vi "HumanExecute.vi"(8 "error in (no error)":errorcluster) -> (0 "error out":errorcluster)   [LabVIEW 2023]
doc: "Execute for Human\n\ninput:\n error in (cluster)\n\noutput:\n error out (cluster)"
uses:
  Arm/ArmPositionPreset.ctl
  Arm/ArmGamePiecePreset.ctl
  <vilib>/Rock Robotics/WPI/Joystick/XBox Buttons Indexer.ctl
  <vilib>/Rock Robotics/WPI/Joystick/XBox Axes Indexer.ctl
  <vilib>/Rock Robotics/WPI/ThirdParty/JAS_Junk/TrajLib/Timer_New.vi
  Claw/ClawGlobal.vi
  <vilib>/Utility/semaphor.llb/Obtain Semaphore Reference.vi
  <vilib>/Rock Robotics/WPI/ThirdParty/JAS_Junk/TrajLib/Timer_Reset.vi
  <vilib>/Rock Robotics/WPI/ThirdParty/JAS_Junk/TrajLib/Timer_Start.vi
  <vilib>/Rock Robotics/WPI/ThirdParty/JAS_Junk/TrajLib/Timer_HasPeriodPassedOnce.vi
  <vilib>/Rock Robotics/WPI/ThirdParty/JAS_Junk/TrajLib/Timer_Stop.vi
  <vilib>/Rock Robotics/WPI/ThirdParty/JAS_Junk/TrajLib/Trajectory_Library.lvlib
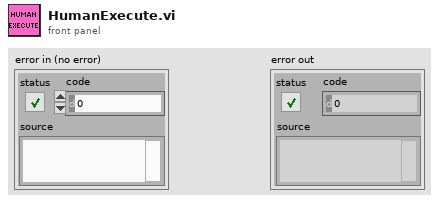
[diagram p1: front panel]
types:
  T1 = typedef "ArmPositionPreset.ctl" = enum16{"Upper", "Lower", "Middle", "Home", "Shelf", "Floor", "HalfFloor", "HalfHome"}
  T2 = typedef "ArmGamePiecePreset.ctl" = enum16{"Cube", "Cone"}
  T3 = typedef "XBox Buttons Indexer.ctl" = enum16{"A", "B", "X", "Y", "Left Bumper", "Right Bumper", "Back", "Start", "Left Joystick", "Right Joystick"}
  T4 = typedef "XBox Axes Indexer.ctl" = enum16{"Left X", "Left Y", "Left Trigger", "Right Trigger", "Right X", "Right Y"}
  T5 = typedef "WPI_JoystickDevRef.ctl" = cluster{"Device":T6}
  T6 = typedef "WPI_JoystickDeviceEnum.ctl" = enum16{"USB 0", "USB 1", "USB 2", "USB 3", "USB 4", "USB 5"}
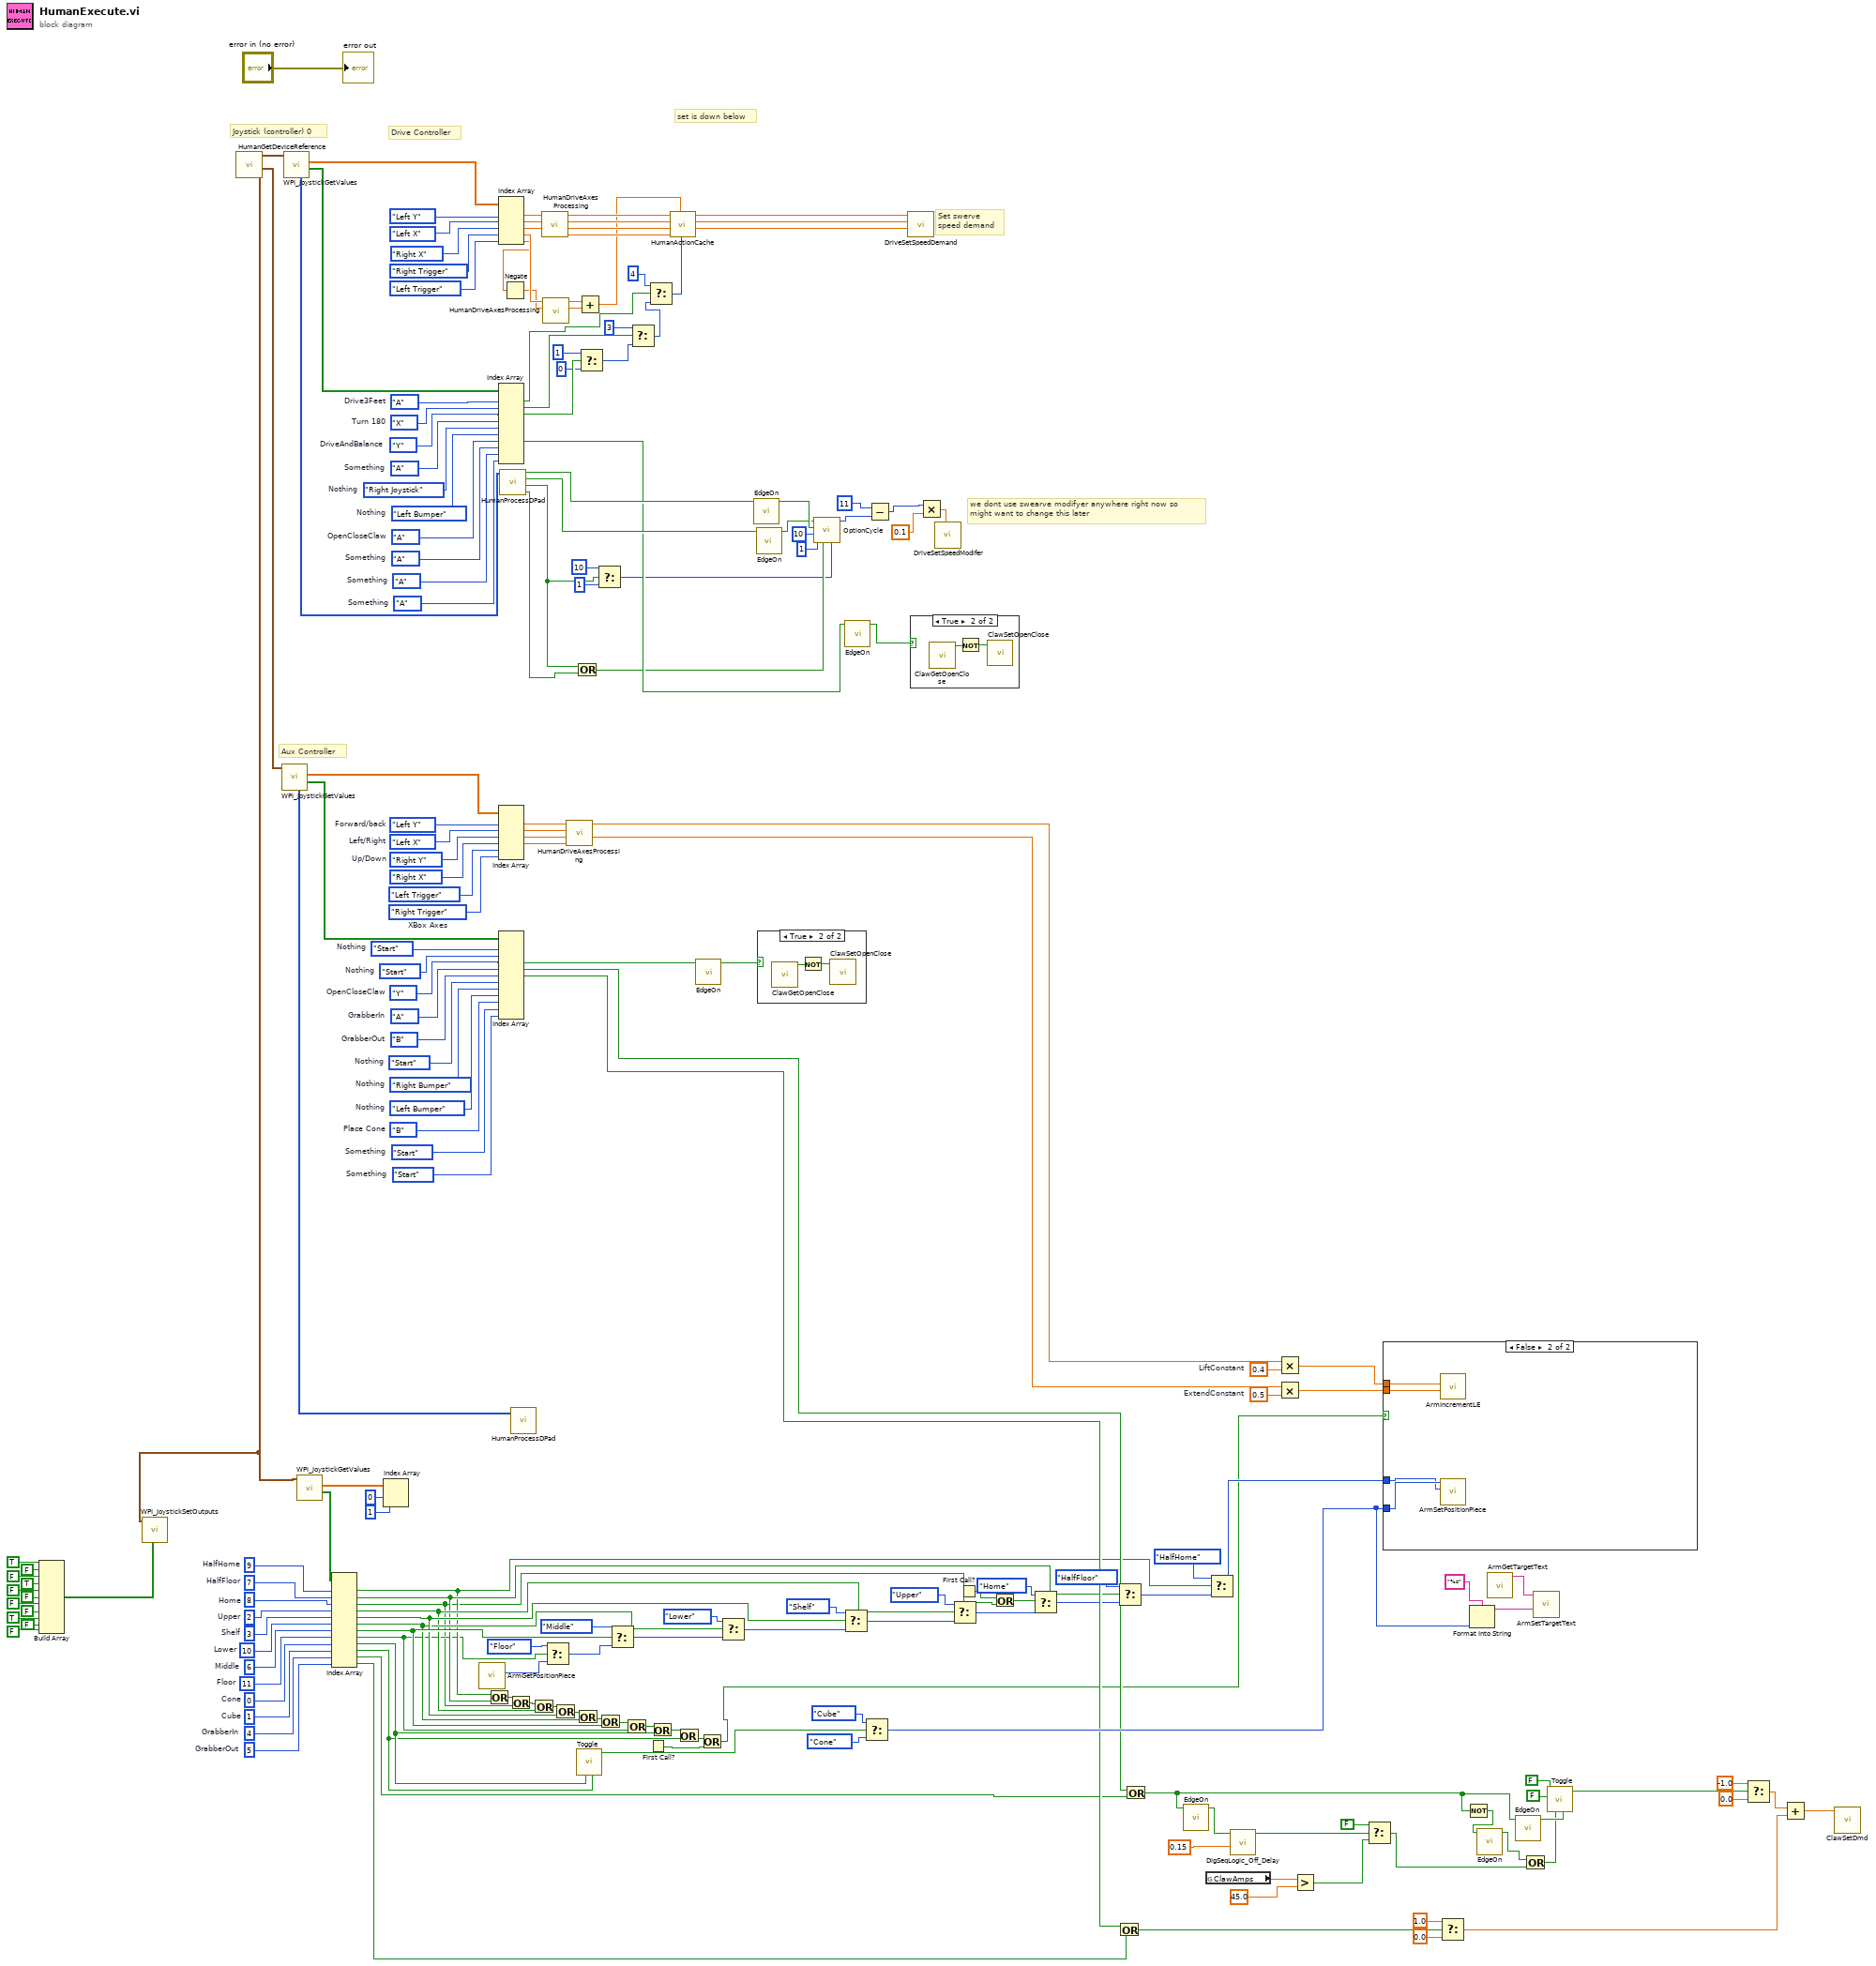
[diagram p0: block diagram]
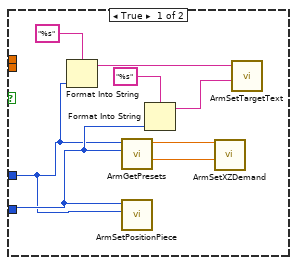
[diagram p3: hidden frame]
diagram:
  w58 = 9  # HalfHome
  w59 = 7  # HalfFloor
  w96 = 8  # Home
  w103 = 0.4  # LiftConstant
  w104 = 0.5  # ExtendConstant
  w116 = 5  # GrabberOut
  w117 = 4  # GrabberIn
  w118 = 1  # Cube
  w119 = 0  # Cone
  w120 = 11  # Floor
  w121 = 6  # Middle
  w122 = 10  # Lower
  w123 = 3  # Shelf
  w124 = 2  # Upper
  w135 = XBox_Buttons_Indexer."Start"  # Something
  w136 = XBox_Buttons_Indexer."Start"  # Something
  w137 = XBox_Buttons_Indexer."B"  # Place Cone
  w138 = XBox_Buttons_Indexer."Left Bumper"  # Nothing
  w139 = XBox_Buttons_Indexer."Right Bumper"  # Nothing
  w140 = XBox_Buttons_Indexer."Start"  # Nothing
  w145 = XBox_Buttons_Indexer."B"  # GrabberOut
  w148 = XBox_Buttons_Indexer."A"  # GrabberIn
  w149 = XBox_Buttons_Indexer."Y"  # OpenCloseClaw
  w150 = XBox_Buttons_Indexer."Start"  # Nothing
  w151 = XBox_Buttons_Indexer."Start"  # Nothing
  w141 = XBox_Axes_Indexer."Right Trigger"  # XBox Axes
  w144 = XBox_Axes_Indexer."Right Y"  # Up/Down
  w152 = XBox_Axes_Indexer."Left X"  # Left/Right
  w153 = XBox_Axes_Indexer."Left Y"  # Forward/back
  w179 = XBox_Buttons_Indexer."A"  # Something
  w180 = XBox_Buttons_Indexer."A"  # Something
  w181 = XBox_Buttons_Indexer."A"  # Something
  w182 = XBox_Buttons_Indexer."A"  # OpenCloseClaw
  w183 = XBox_Buttons_Indexer."Left Bumper"  # Nothing
  w190 = XBox_Buttons_Indexer."Right Joystick"  # Nothing
  w191 = XBox_Buttons_Indexer."A"  # Something
  w193 = XBox_Buttons_Indexer."Y"  # DriveAndBalance
  w194 = XBox_Buttons_Indexer."X"  # Turn 180
  w195 = XBox_Buttons_Indexer."A"  # Drive3Feet
  # "set is down below"
  # "we dont use swearve modifyer anywhere right now so\nmight want to change this later"
  # "Aux Controller"
  # "Set swerve\nspeed demand"
  # "Joystick (controller) 0"
  # "Drive Controller"
  n1 = Build Array(TRUE, FALSE ("element"), FALSE ("element"), TRUE ("element"), FALSE ("element"), FALSE ("element"), FALSE ("element"), FALSE ("element"), TRUE ("element"), FALSE ("element"), FALSE ("element")) -> (w173:bool[])
  n2 = call "HumanGetDeviceReference.vi"() -> ("ButtonBoard"=w174:T5, "Aux Joy"=w197:T5, "Driver Joy"=w198:T5)  [unwired: 9 in]
  n3 = call <vilib>:"WPI_JoystickSetOutputs.vi"("Outputs"=w173, "JoystickDevRef"=w174) -> ()  [unwired: 8 in, 2 out]
  n4 = call <vilib>:"WPI_JoystickGetValues.vi"("JoystickDevRef"=w197) -> ("Buttons"=w146:bool[], "Axes"=w147:dbl[], "POVs"=w134:i16[])  [unwired: 6 in, 2 out]
  n5 = call <vilib>:"WPI_JoystickGetValues.vi"("JoystickDevRef"=w198) -> ("Buttons"=w196:bool[], "Axes"=w202:dbl[], "POVs"=w192:i16[])  [unwired: 6 in, 2 out]
  n6 = call <vilib>:"WPI_JoystickGetValues.vi"("JoystickDevRef"=w174) -> ("Buttons"=w128:bool[], "Axes"=w127:dbl[])  [unwired: 6 in, 3 out]
  n7 = Index Array "Index Array"(array=w128, index #1=w58, index #2=w59, index #3=w96, index #4=w124, index #5=w123, index #6=w122, index #7=w121, index #8=w120, index #9=w119, index #10=w118, index #11=w117, index #12=w116) -> (element #1=w60:bool, element #2=w61:bool, element #3=w35:bool, element #4=w93:bool, element #5=w108:bool, element #6=w102:bool, element #7=w109:bool, element #8=w55:bool, element #9=w84:bool, element #10=w83:bool, element #11=w53:bool, element #12=w71:bool)
  n8 = Index Array "Index Array"(array=w127, index #1=0 ("index"), index #2=1 ("index")) -> ()  [unwired: 2 out]
  n9 = call "ArmGetPositionPiece.vi"() -> ("Position"=w54:T1)  [unwired: 10 in, 1 out]
  n10 = Or(x=w60, y=w61) -> (x .or. y?=w63:bool)
  n11 = Index Array(array=w202, index #1=XBox_Axes_Indexer."Left Y" ("XBox Axes"), index #2=XBox_Axes_Indexer."Left X" ("XBox Axes"), index #3=XBox_Axes_Indexer."Right X" ("XBox Axes"), index #4=XBox_Axes_Indexer."Right Trigger" ("XBox Axes"), index #5=XBox_Axes_Indexer."Left Trigger" ("XBox Axes")) -> (element #1=w188:dbl, element #2=w187:dbl, element #3=w186:dbl, element #4=w159:dbl, element #5=w158:dbl)
  n12 = Index Array(array=w196, index #1=w195, index #2=w194, index #3=w193, index #4=w191, index #5=w190, index #6=w183, index #7=w182, index #8=w181, index #9=w180, index #10=w179) -> (element #1=w2:bool, element #2=w164:bool, element #3=w184:bool, element #7=w175:bool)  [unwired: 6 out]
  n13 = Index Array(array=w147, index #1=w153, index #2=w152, index #3=w144, index #4=XBox_Axes_Indexer."Right X" ("XBox Axes"), index #5=XBox_Axes_Indexer."Left Trigger", index #6=w141) -> (element #1=w133:dbl, element #2=w132:dbl, element #3=w131:dbl, element #4=w130:dbl)  [unwired: 2 out]
  n14 = Index Array "Index Array"(array=w146, index #1=w151, index #2=w150, index #3=w149, index #4=w148, index #5=w145, index #6=w140, index #7=w139, index #8=w138, index #9=w137, index #10=w136, index #11=w135) -> (element #3=w107:bool, element #4=w70:bool, element #5=w69:bool)  [unwired: 8 out]
  n15 = call "HumanProcessDPad.vi"("POV"=w192) -> ("Right"=w171:bool, "Left"=w170:bool, "Down"=w177:bool, "Up"=w178:bool)  [unwired: 7 in]
  n16 = Negate(x=w158) -> (-x=w157:dbl)
  n17 = Or(x=w63, y=w35) -> (x .or. y?=w62:bool)
  n18 = call "HumanProcessDPad.vi"("POV"=w134) -> ()  [unwired: 7 in, 4 out]
  n19 = Or(x=w62, y=w93) -> (x .or. y?=w94:bool)
  n20 = call "HumanDriveAxesProcessing.vi"("Right Y"=w186, "Left X"=w187, "Left Y"=w188) -> ("Right X"=w185:dbl, "Right Y"=w154:dbl, "Left X"=w160:dbl, "Left Y"=w9:dbl)  [unwired: 5 in]
  n21 = call "HumanDriveAxesProcessing.vi"("Left X"=w157, "Left Y"=w159) -> ("Left X"=w155:dbl, "Left Y"=w156:dbl)  [unwired: 6 in, 2 out]
  n22 = Select(t=ArmPositionPreset."Floor" ("Position"), s=w55, f=w54) -> (s? t:f=w57:T1)
  n23 = Or(x=w94, y=w108) -> (x .or. y?=w112:bool)
  n24 = call "HumanDriveAxesProcessing.vi"("Right X"=w130, "Right Y"=w131, "Left X"=w132, "Left Y"=w133) -> ("Right Y"=w105:dbl, "Left Y"=w106:dbl)  [unwired: 4 in, 2 out]
  n25 = Or(x=w170, y=w171) -> (x .or. y?=w172:bool)
  n26 = Or(x=w112, y=w102) -> (x .or. y?=w111:bool)
  n27 = call "Toggle.vi"("SetTrue"=w83, "SetFalse"=w84) -> ("Toggled"=w99:bool)  [unwired: 9 in]
  n28 = Add(x=w156, y=w155) -> (x+y=w8:dbl)
  n29 = Select(t=1, s=w184, f=0) -> (s? t:f=w165:i32)
  n30 = Select(t=10 ("MinValue"), s=w170, f=1) -> (s? t:f=w167:i32)
  n31 = Or(x=w111, y=w109) -> (x .or. y?=w110:bool)
  n32 = Select(t=ArmPositionPreset."Middle" ("Position"), s=w109, f=w57) -> (s? t:f=w114:T1)
  n33 = Or(x=w110, y=w55) -> (x .or. y?=w86:bool)
  n34 = Select(t=3, s=w164, f=w165) -> (s? t:f=w3:i32)
  n35 = First Call?() -> (First Call?: T/F=w32:bool)
  n36 = Select(t=4, s=w2, f=w3) -> (s? t:f=w4:i32)
  n37 = Or(x=w86, y=w84) -> (x .or. y?=w85:bool)
  n38 = call "HumanActionCache.vi"("State"=w4, "Rotation"=w8, "Right X"=w185, "Right Y"=w154, "Left X"=w160, "Left Y"=w9) -> ("AMotorDemand"=w7:dbl, "YMotorDemand"=w6:dbl, "XMotorDemand"=w5:dbl)  [unwired: 3 in]
  n39 = Or(x=w85, y=w83) -> (x .or. y?=w33:bool)
  n40 = call "EdgeOn.vi"("Current State"=w107) -> ("Edge On Found"=w129:bool)  [unwired: 10 in]
  n41 = Or(x=w33, y=w32) -> (x .or. y?=w31:bool)
  n42 = Select(t=ArmPositionPreset."Lower" ("Position"), s=w102, f=w114) -> (s? t:f=w115:T1)
  n43 = call "EdgeOn.vi"("Current State"=w178) -> ("Edge On Found"=w13:bool)  [unwired: 10 in]
  n44 = call "EdgeOn.vi"("Current State"=w177) -> ("Edge On Found"=w12:bool)  [unwired: 10 in]
  n45 = case shown="True" w129 {
    frame False {
    }
    frame True {
      n46 = call "ClawGetOpenClose.vi"() -> ("Open?"=w204:bool)  [unwired: 11 in]
      n47 = Not(x=w204) -> (.not. x?=w203:bool)
      n48 = call "ClawSetOpenClose.vi"("Open?"=w203) -> ()  [unwired: 11 in]
    }
  }
  n49 = call "OptionCycle.vi"("ValuetoSet"=w167, "SetValue"=w172, "MinValue"=1, "MaxValue"=10, "BackwardsInput"=w13, "ForwardInput"=w12) -> ("CycleNum"=w16:i32)  [unwired: 5 in]
  n50 = Select(t=ArmPositionPreset."Shelf" ("Position"), s=w108, f=w115) -> (s? t:f=w113:T1)
  n51 = call "EdgeOn.vi"("Current State"=w175) -> ("Edge On Found"=w19:bool)  [unwired: 10 in]
  n52 = Select(t=ArmGamePiecePreset."Cube" ("Game Piece"), s=w99, f=ArmGamePiecePreset."Cone" ("Game Piece")) -> (s? t:f=w87:T2)
  n53 = Subtract(x=11, y=w16) -> (x-y=w14:i32)
  n54 = call "DriveSetSpeedDemand.vi"("ASpeedDemand (d/s)"=w7, "YSpeedDemand (ft/s)"=w6, "XSpeedDemand (ft/s)"=w5) -> ()  [unwired: 9 in]
  n55 = case shown="True" w19 {
    frame False {
    }
    frame True {
      n56 = call "ClawGetOpenClose.vi"() -> ("Open?"=w206:bool)  [unwired: 11 in]
      n57 = Not(x=w206) -> (.not. x?=w205:bool)
      n58 = call "ClawSetOpenClose.vi"("Open?"=w205) -> ()  [unwired: 11 in]
    }
  }
  n59 = Multiply(x=w14, y=0.1) -> (x*y=w17:dbl)
  n60 = call "DriveSetSpeedModifer.vi"("SpeedModifer"=w17) -> ()  [unwired: 11 in]
  n61 = Select(t=ArmPositionPreset."Upper" ("Position"), s=w93, f=w113) -> (s? t:f=w95:T1)
  n62 = First Call?() -> (First Call?: T/F=w36:bool)
  n63 = Or(x=w36, y=w35) -> (x .or. y?=w34:bool)
  n64 = Select(t=ArmPositionPreset."Home" ("Position"), s=w34, f=w95) -> (s? t:f=w68:T1)
  n65 = Or(x=w69, y=w71) -> (x .or. y?=w72:bool)
  n66 = Select(t=ArmPositionPreset."HalfFloor", s=w61, f=w68) -> (s? t:f=w67:T1)
  n67 = Or(x=w70, y=w53) -> (x .or. y?=w42:bool)
  n68 = call "EdgeOn.vi"("Current State"=w42) -> ("Edge On Found"=w41:bool)  [unwired: 10 in]
  n69 = global read "ClawGlobal.vi" "ClawAmps"() -> (w48:dbl)
  n70 = Select(t=ArmPositionPreset."HalfHome", s=w60, f=w67) -> (s? t:f=w64:T1)
  n71 = call <vilib>:"DigSeqLogic_Off_Delay.vi"("Delay"=0.15 ("Off Delay Tme\nSeconds"), "Input"=w41) -> ("Output"=w40:bool)  [unwired: 8 in, 1 out]
  n72 = Multiply(x=w106, y=w103) -> (x*y=w100:dbl)
  n73 = Multiply(x=w105, y=w104) -> (x*y=w101:dbl)
  n74 = Greater?(x=w48, y=45.0) -> (0:w39:bool)
  n75 = Select(t=FALSE, s=w40, f=w39) -> (s? t:f=w37:bool)
  n76 = case shown="False" w31 {
    tunnel: w101 -> [_ w218]
    tunnel: w100 -> [_ w217]
    tunnel: w87 -> [w208 w216]
    tunnel: w64 -> [w207 w215]
    frame True {
      n77 = Format Into String(format string="%s", w207) -> (resulting string=w212:string)  [unwired: 2 in, 1 out]
      n78 = call "ArmGetPresets.vi"("Game Piece"=w208, "Position"=w207) -> ("z"=w213:dbl, "x"=w214:dbl)  [unwired: 8 in]
      n79 = call "ArmSetPositionPiece.vi"("Position"=w207, "Game Piece"=w208) -> ()  [unwired: 10 in]
      n80 = Format Into String(format string="%s", w208) -> (resulting string=w209:string)  [unwired: 2 in, 1 out]
      n81 = call "ArmSetXZDemand.vi"("SetZ"=w213, "SetX"=w214) -> ()  [unwired: 10 in]
      n82 = call "ArmSetTargetText.vi"("TargetGamePiece"=w209, "TargetArmPosition"=w212) -> ()  [unwired: 10 in]
    }
    frame False {
      n83 = call "ArmIncrementLE.vi"("AddE"=w218, "AddL"=w217) -> ()  [unwired: 10 in]
      n84 = call "ArmSetPositionPiece.vi"("Position"=w215, "Game Piece"=w216) -> ()  [unwired: 10 in]
    }
  }
  n85 = Select(t=1.0, s=w72, f=0.0) -> (s? t:f=w78:dbl)
  n86 = Not(x=w42) -> (.not. x?=w44:bool)
  n87 = Format Into String(format string="%s", w87) -> (resulting string=w82:string)  [unwired: 2 in, 1 out]
  n88 = call "EdgeOn.vi"("Current State"=w44) -> ("Edge On Found"=w45:bool)  [unwired: 10 in]
  n89 = call "ArmGetTargetText.vi"() -> ("TargetArmPosition"=w80:string)  [unwired: 10 in, 1 out]
  n90 = call "EdgeOn.vi"("Current State"=w42) -> ("Edge On Found"=w52:bool)  [unwired: 10 in]
  n91 = Or(x=w45, y=w37) -> (x .or. y?=w46:bool)
  n92 = call "ArmSetTargetText.vi"("TargetGamePiece"=w82, "TargetArmPosition"=w80) -> ()  [unwired: 10 in]
  n93 = call "Toggle.vi"("SetTrue"=w52, "SetFalse"=w46, "InitialState"=FALSE, "FlashInput"=FALSE) -> ("Toggled"=w51:bool)  [unwired: 7 in]
  n94 = Select(t=-1.0, s=w51, f=0.0) -> (s? t:f=w79:dbl)
  n95 = Add(x=w79, y=w78) -> (x+y=w77:dbl)
  n96 = call "ClawSetDmd.vi"("ClawDemand"=w77) -> ()  [unwired: 11 in]
  "error out" <- "error in (no error)"
